vi "BonOMM-SAOMM.Test.vi"() -> ()   [LabVIEW 2011] (continued)
                            n700 = local read "properties.ini"() -> (w3967:path)
                            n701 = call "SerialCommError.vi"("VISA IN"=w3963, "error IN"=w3964) -> ("VISA OUT"=w3978:refnum<visa-resource-name>, "Error"=w3966:bool, "error OUT"=w3958:errorcluster)  [unwired: 11 in]
                            n702 = Not(x=w3966) -> (.not. x?=w3959:bool)
                            n703 = call <vilib>:"Open Config Data.vi"("configuration file path"=w3967) -> ("error out"=w3976:errorcluster, "refnum"=w3977:T24)  [unwired: 8 in, 1 out]
                            n704 = local write "TCS VRN"(w3978) -> ()
                            n705 = local write "TCS Error"(w3958) -> ()
                            n706 = case shown="True" w3959 {
                              tunnel: [TRUE ("Boolean") w4021] -> w3961
                              frame False {
                              }
                              frame True {
                                n707 = Two Button Dialog(message="La connexion TCP/IP semble fonctionner.\nDésirez-vous vraiment la réinitialiser ?" ("T button name (\"OK\")"), 1:"Non" ("F button name (\"Cancel\")"), 2:"Oui" ("T button name (\"OK\")")) -> (T button?=w4021:bool)
                              }
                            }
                            n708 = call-poly <vilib>:"Read Key.vi"("section"=w3971, "error in (no error)"=w3976, "key"="TCS-IP" ("name or relative path"), "refnum"=w3977) -> ("error out"=w3974:errorcluster, "value"=w3962:string, "refnum out"=w3975:T24)  [unwired: 4 in, 1 out]
                            n709 = call-poly <vilib>:"Read Key.vi"("section"=w3971, "error in (no error)"=w3974, "key"="TCS-PN" ("name or relative path"), "refnum"=w3975) -> ("error out"=w3972:errorcluster, "value"=w3968:u32, "refnum out"=w3973:T24)  [unwired: 4 in, 1 out]
                            n710 = call <vilib>:"Close Config Data.vi"("error in (no error)"=w3972, "refnum"=w3973) -> ()  [unwired: 8 in, 2 out]
                            n711 = case shown="True" w3961 {
                              tunnel: w3968 -> [_ w3984]
                              tunnel: w3962 -> [_ w3985]
                              tunnel: w3960 -> [_ w3986]
                              frame False {
                              }
                              frame True {
                                n712 = flat-sequence {
                                tunnel: w3986 -> [w3993]
                                tunnel: [refnum<visa-resource-name> "-1" ("Table VRN")] -> w3981
                                tunnel: [w3990] -> w3980
                                tunnel: w3981 -> [w3997]
                                tunnel: w3980 -> [w3996]
                                tunnel: [w3994] -> w3979
                                tunnel: w3979 -> [_]
                                tunnel: w3985 -> [w4004]
                                tunnel: w3984 -> [w4003]
                                tunnel: [w4002] -> w3983
                                tunnel: [w4001] -> w3982
                                tunnel: [w4015] -> w3988
                                tunnel: [w4014] -> w3987
                                tunnel: w3982 -> [_]
                                tunnel: w3983 -> [w4009]
                                tunnel: w3988 -> [w4017]
                                tunnel: w3987 -> [w4016]
                                frame #0 {
                                w3989 = TRUE ("TCS R actif")
                                n713 = local write "ReconnectionMute"(w3989) -> ()
                                n714 = local read "TCS VRN"() -> (w3990:refnum<visa-resource-name>)
                                n715 = call "TCS-Wait4Flag.vi"("Raise Flag ?"=TRUE, "Ctl Refnum IN"=w3993) -> ()  [unwired: 8 in, 2 out]
                                "TCSMute" <- w3989
                                }
                                frame #1 {
                                n716 = local write "TCS VRN"(w3997) -> ()
                                n717 = Type Cast(type=refnum<k5> refnum ("connection ID out"), x=w3996) -> (*(type *) &x=w3998:refnum<k5>)
                                n718 = TCP Close Connection(connection ID=w3998) -> (error out=w3994:errorcluster)  [unwired: 2 in, 1 out]
                                }
                                frame #2 {
                                n719 = Wait (ms)(milliseconds to wait=u32 1000) -> ()  [unwired: 1 out]
                                }
                                frame #3 {
                                n720 = To Unsigned Word Integer(number=w4003) -> (unsigned 16bit integer=w4005:u16)
                                n721 = local write "TCS actif"(FALSE ("TCS R actif")) -> ()
                                n722 = TCP Open Connection(address=w4004, remote port or service name=w4005) -> (connection ID=w4002:refnum<k5>, error out=w4001:errorcluster)  [unwired: 3 in]
                                }
                                frame #4 {
                                # "Doit-on fermer la \nconnexion d'abord ?"
                                n723 = Type Cast(type="", x=w4009) -> (*(type *) &x=w4012:string)
                                n724 = control-ref of="TCS actif"() -> (w4006:refnum<vi>)
                                n725 = Type Cast(type=refnum<visa-resource-name> "-1" ("Table VRN"), x=w4012) -> (*(type *) &x=w4010:refnum<visa-resource-name>)
                                n726 = call "EXCOM-25-EQ.vi"("VISA resource name"=w4010, "Bool Refnum"=w4006) -> ("VISA resource name dup"=w4008:refnum<visa-resource-name>, "Error OUT"=w4007:errorcluster)  [unwired: 3 in, 13 out]
                                n727 = call "SerialCommError.vi"("VISA IN"=w4008, "error IN"=w4007) -> ("VISA OUT"=w4015:refnum<visa-resource-name>, "error OUT"=w4014:errorcluster)  [unwired: 11 in, 1 out]
                                }
                                frame #5 {
                                n728 = case shown="Error" w4016 {
                                frame No Error {
                                }
                                frame Error {
                                n729 = One Button Dialog(message="La communication avec le TCS ne semble toujours pas foncitonner.\nVérifiez les connexions et les paramètres puis recommencez." ("T button name (\"OK\")")) -> ()  [unwired: 1 in, 1 out]
                                }
                                }
                                n730 = local write "TCS Error"(w4016) -> ()
                                n731 = local write "TCS VRN"(w4017) -> ()
                                }
                                frame #6 {
                                w4019 = FALSE
                                n732 = local write "ReconnectionMute"(w4019) -> ()
                                n733 = local write "TCSMute"(w4019) -> ()
                                }
                                }
                              }
                            }
                          }
                        }
                      }
                      frame "com_Caméra de référence" {
                        n734 = local read "exptime"() -> (w4027:dbl)
                        n735 = local read "MessageType"() -> (w4032:cluster{string[], u32[]})
                        n736 = control-ref of="PrAMS actif"() -> (w4036:refnum<vi>)
                        n737 = local read "Signature"() -> (w4035:u32)
                        n738 = control-ref of="PrAMS-ACK"() -> (w4037:refnum<vi>)
                        n739 = local read "PrAMS VRN"() -> (w4038:refnum<visa-resource-name>)
                        n740 = expression code="x*1000"(w4027) -> (w4030:dbl)
                        n741 = To Unsigned Long Integer(number=w4030) -> (unsigned 32bit integer=w4029:u32)
                        n742 = call-poly "SAOMM-Num2littleEndian.vi"("Number"=w4029) -> ("LiitleEndianedData"=w4028:u8[])  [unwired: 14 in]
                        n743 = call "SAOMM-SendSET.vi"("PRAMMS-COMM IN"=w4038, "Active Refnum"=w4036, "PrAMS-ACK"=w4037, "Signature"=w4035, "Error IN"=errorcluster {"status"=FALSE, "code"=0, "source"=""} ("PRAMMS Error"), "MessageType"=w4032, "Active SET"="emtSetImageExposureTime", "Value (little endianed byte array)"=w4028) -> ("Error"=w4026:bool, "Error OUT"=w4034:errorcluster)  [unwired: 4 in, 2 out]
                        n744 = local write "PrAMS Error"(w4034) -> ()
                        n745 = Not(x=w4026) -> (.not. x?=w4025:bool)
                        n746 = case shown="True" w4025 {
                          tunnel: [TRUE ("Boolean") w4041] -> w4039
                          frame False {
                          }
                          frame True {
                            n747 = Two Button Dialog(message="La connexion TCP/IP semble fonctionner.\nDésirez-vous vraiment la réinitialiser ?" ("T button name (\"OK\")"), 1:"Non" ("F button name (\"Cancel\")"), 2:"Oui" ("T button name (\"OK\")")) -> (T button?=w4041:bool)
                          }
                        }
                        n748 = case shown="True" w4039 {
                          frame False {
                          }
                          frame True {
                            n749 = flat-sequence {
                              tunnel: [w4046] -> w4045
                              tunnel: w4045 -> [_]
                              frame #0 {
                                n750 = local read "PrAMS VRN"() -> (w4048:refnum<visa-resource-name>)
                                n751 = Type Cast(type=refnum<k5> refnum ("connection ID"), x=w4048) -> (*(type *) &x=w4047:refnum<k5>)
                                n752 = TCP Close Connection(connection ID=w4047) -> (error out=w4046:errorcluster)  [unwired: 2 in, 1 out]
                              }
                              frame #1 {
                                n753 = local read "properties.ini"() -> (w4058:path)
                                n754 = local read "path_config"() -> (w4051:path)
                                n755 = Build Path(base path=w4051, name or relative path=path "command.ini" ("command.ini")) -> (appended path=w4050:path)
                                n756 = call <vilib>:"Open Config Data.vi"("create file if necessary (T)"=FALSE, "configuration file path"=w4058) -> ("error out"=w4056:errorcluster, "refnum"=w4055:T24)  [unwired: 7 in, 1 out]
                                n757 = local read "Signature"() -> (w4067:u32)
                                n758 = call-poly <vilib>:"Read Key.vi"("section"="communications" ("key"), "error in (no error)"=w4056, "key"="PRAMMS-IP", "refnum"=w4055) -> ("error out"=w4062:errorcluster, "value"=w4054:string, "refnum out"=w4061:T24)  [unwired: 4 in, 1 out]
                                n759 = call <vilib>:"Close Config Data.vi"("error in (no error)"=w4062, "refnum"=w4061) -> ()  [unwired: 8 in, 2 out]
                                n760 = call "SAOMM-connect.vi"("IP"=w4054, "Port"=u16 10010, "Signature"=w4067, "Command.ini"=w4050) -> ("connection ID"=w4064:refnum<k5>, "Error OUT"=w4053:errorcluster)  [unwired: 7 in, 3 out]
                                n761 = disable-structure shown="Disabled" {
                                disable-tunnel: w4053 -> [w4069 _]
                                frame Disabled {
                                n762 = case shown="Error" w4069 {
                                frame No Error {
                                }
                                frame Error {
                                n763 = One Button Dialog(message="Erreur lors de la connexion\nà l'hexapode-console.") -> ()  [unwired: 1 in, 1 out]
                                }
                                }
                                }
                                frame Enabled {
                                }
                                }
                                n764 = local read "PrAMS VRN"() -> (w4066:refnum<visa-resource-name>)
                                n765 = local write "PrAMS Error"(w4053) -> ()
                                n766 = Type Cast(type=w4054, x=w4064) -> (*(type *) &x=w4063:string)
                                n767 = Type Cast(type=w4066, x=w4063) -> (*(type *) &x=w4065:refnum<visa-resource-name>)
                                n768 = local write "PrAMS VRN"(w4065) -> ()
                              }
                            }
                          }
                        }
                      }
                      frame "com_Tables de guidage" {
                        n769 = flat-sequence {
                          frame #0 {
                            w4072 = TRUE
                            n770 = local write "Sync_Ready"(FALSE ("Sync_Ready")) -> ()
                            "TableMute" <- w4072
                            "ReconnectionMute" <- w4072
                          }
                          frame #1 {
                            w4087 = "communications" ("name or relative path")
                            n771 = local read "Table VRN"() -> (w4076:refnum<visa-resource-name>)
                            n772 = local read "properties.ini"() -> (w4080:path)
                            n773 = control-ref of="Table actif"() -> (w4074:refnum<vi>)
                            n774 = local read "ActiveStages"() -> (w4073:string[])
                            n775 = call "Newmark-Status-All.vi"("Table VRN IN"=w4076, "Bool Refnum"=w4074, "StageTag"=w4073) -> ("Table VRN OUT"=w4077:refnum<visa-resource-name>, "Error OUT"=w4075:errorcluster)  [unwired: 4 in, 11 out]
                            n776 = call <vilib>:"Open Config Data.vi"("configuration file path"=w4080) -> ("error out"=w4092:errorcluster, "refnum"=w4093:T24)  [unwired: 8 in, 1 out]
                            n777 = call "SerialCommError.vi"("VISA IN"=w4077, "error IN"=w4075) -> ("VISA OUT"=w4094:refnum<visa-resource-name>, "Error"=w4078:bool)  [unwired: 11 in, 1 out]
                            n778 = case shown="True" w4078 {
                              selector: w4078 -> [_ w4107]
                              tunnel: [w4103 w4107] -> w4079
                              frame False {
                                n779 = Two Button Dialog(message="La communication avec les tables semble bonne.\nDésirez-vous vraiment le réinitialiser ?" ("T button name (\"OK\")"), 1:"Non" ("F button name (\"Cancel\")"), 2:"Oui" ("T button name (\"OK\")")) -> (T button?=w4103:bool)
                              }
                              frame True {
                              }
                            }
                            n780 = call-poly <vilib>:"Read Key.vi"("section"=w4087, "error in (no error)"=w4092, "key"="tablevrn" ("name or relative path"), "refnum"=w4093) -> ("error out"=w4090:errorcluster, "value"=w4083:string, "refnum out"=w4091:T24)  [unwired: 4 in, 1 out]
                            n781 = local write "Table VRN"(w4094) -> ()
                            n782 = call-poly <vilib>:"Read Key.vi"("section"=w4087, "error in (no error)"=w4090, "key"="tablespd" ("name or relative path"), "refnum"=w4091) -> ("error out"=w4088:errorcluster, "value"=w4084:u32, "refnum out"=w4089:T24)  [unwired: 4 in, 1 out]
                            n783 = Type Cast(type=refnum<visa-resource-name> "-1" ("TCS R VRN"), x=w4083) -> (*(type *) &x=w4081:refnum<visa-resource-name>)
                            n784 = call <vilib>:"Close Config Data.vi"("error in (no error)"=w4088, "refnum"=w4089) -> ()  [unwired: 8 in, 2 out]
                            n785 = case shown="True" w4079 {
                              tunnel: w4084 -> [_ w4100]
                              tunnel: w4081 -> [_ w4099]
                              frame False {
                              }
                              frame True {
                                n786 = local write "Table Baud rate"(w4100) -> ()
                                n787 = control-ref of="Table actif"() -> (w4097:refnum<vi>)
                                n788 = local read "ActiveStages"() -> (w4098:string[])
                                n789 = call "Newmark-Initialize.vi"("VISA resource name"=w4099, "ActiveStages"=w4098, "baud rate"=w4100, "Timeout"=u32 1000, "Bool Refnum"=w4097) -> ("VISA resource name out"=w4101:refnum<visa-resource-name>, "Error OUT"=w4095:errorcluster)  [unwired: 8 in, 1 out]
                                n790 = local write "Table Error"(w4095) -> ()
                                n791 = case shown="No Error" w4095 {
                                frame No Error {
                                }
                                frame Error {
                                n792 = One Button Dialog(message="La communication avec les tables  ne semble toujours pas foncitonner.\nVérifiez les connexions et les paramètres puis recommencez." ("T button name (\"OK\")")) -> ()  [unwired: 1 in, 1 out]
                                }
                                }
                                n793 = local write "Table VRN"(w4101) -> ()
                              }
                            }
                          }
                          frame #2 {
                            w4109 = FALSE
                            n794 = local write "ReconnectionMute"(w4109) -> ()
                            n795 = local write "Sync_Ready"(TRUE ("Sync_Ready")) -> ()
                            n796 = local write "TableMute"(w4109) -> ()
                          }
                        }
                      }
                      frame "com_Secondaire Actif" {
                        (unwired) FALSE
                        w4119 = "communications" ("name or relative path")
                        n797 = local read "properties.ini"() -> (w4114:path)
                        n798 = call <vilib>:"Open Config Data.vi"("configuration file path"=w4114) -> ("error out"=w4124:errorcluster, "refnum"=w4125:T24)  [unwired: 8 in, 1 out]
                        n799 = One Button Dialog(message="À compléter ...") -> ()  [unwired: 1 in, 1 out]
                        n800 = call-poly <vilib>:"Read Key.vi"("section"=w4119, "error in (no error)"=w4124, "key"="PRAMMS-IP" ("name or relative path"), "refnum"=w4125) -> ("error out"=w4122:errorcluster, "value"=w4116:string, "refnum out"=w4123:T24)  [unwired: 4 in, 1 out]
                        n801 = call-poly <vilib>:"Read Key.vi"("section"=w4119, "error in (no error)"=w4122, "key"="PRAMMS-IP" ("name or relative path"), "refnum"=w4123) -> ("error out"=w4120:errorcluster, "value"=w4113:u32, "refnum out"=w4121:T24)  [unwired: 4 in, 1 out]
                        n802 = Type Cast(type=refnum<visa-resource-name> "-1" ("TCS R VRN"), x=w4116) -> (*(type *) &x=w4112:refnum<visa-resource-name>)
                        n803 = call <vilib>:"Close Config Data.vi"("error in (no error)"=w4120, "refnum"=w4121) -> ()  [unwired: 8 in, 2 out]
                        n804 = case shown="True" TRUE {
                          tunnel: w4113 -> [_ _]
                          tunnel: w4112 -> [_ _]
                          frame False {
                          }
                          frame True {
                          }
                        }
                      }
                      frame "com_Lampes de calibration" {
                        n805 = flat-sequence {
                          frame #0 {
                            w4133 = "communications" ("name or relative path")
                            n806 = local read "properties.ini"() -> (w4126:path)
                            n807 = call <vilib>:"Open Config Data.vi"("configuration file path"=w4126) -> ("error out"=w4128:errorcluster, "refnum"=w4127:T24)  [unwired: 8 in, 1 out]
                            n808 = call-poly <vilib>:"Read Key.vi"("section"=w4133, "error in (no error)"=w4128, "key"="calibvrn" ("name or relative path"), "refnum"=w4127) -> ("error out"=w4130:errorcluster, "value"=w4136:string, "refnum out"=w4129:T24)  [unwired: 4 in, 1 out]
                            n809 = call-poly <vilib>:"Read Key.vi"("section"=w4133, "error in (no error)"=w4130, "key"="calibspd" ("name or relative path"), "refnum"=w4129) -> ("error out"=w4132:errorcluster, "value"=w4139:u32, "refnum out"=w4131:T24)  [unwired: 4 in, 1 out]
                            n810 = Type Cast(type=refnum<visa-resource-name> "-1" ("TCS R VRN"), x=w4136) -> (*(type *) &x=w4138:refnum<visa-resource-name>)
                            n811 = call <vilib>:"Close Config Data.vi"("error in (no error)"=w4132, "refnum"=w4131) -> ()  [unwired: 8 in, 2 out]
                            n812 = call-poly "VISA Configure Serial Port"("VISA resource name"=w4138, "timeout (10sec)"=u32 2000, "Enable Termination\nChar (T)"=FALSE ("Enable Termination\nChar (T)"), "baud rate (9600)"=w4139) -> ("VISA resource name out"=w4142:refnum<visa-resource-name>, "error out"=w4143:errorcluster)  [unwired: 10 in]
                            n813 = call "SerialCommError.vi"("VISA IN"=w4142, "error IN"=w4143) -> ("VISA OUT"=w4144:refnum<visa-resource-name>)  [unwired: 11 in, 2 out]
                            n814 = local write "Calib VRN"(w4144) -> ()
                          }
                          frame #1 {
                            n815 = One Button Dialog(message="Le port série des lampes de calibration a été réinitialisé.\n(Aucun test réel car la communication est à sens unique)") -> ()  [unwired: 1 in, 1 out]
                          }
                        }
                      }
                      frame "com_Commandes externes" {
                        (unwired) TRUE
                        n816 = flat-sequence {
                          frame #0 {
                            w4154 = "communications" ("name or relative path")
                            n817 = local read "properties.ini"() -> (w4147:path)
                            n818 = call <vilib>:"Open Config Data.vi"("configuration file path"=w4147) -> ("error out"=w4149:errorcluster, "refnum"=w4148:T24)  [unwired: 8 in, 1 out]
                            n819 = call-poly <vilib>:"Read Key.vi"("section"=w4154, "error in (no error)"=w4149, "key"="excvrn" ("name or relative path"), "refnum"=w4148) -> ("error out"=w4151:errorcluster, "value"=w4157:string, "refnum out"=w4150:T24)  [unwired: 4 in, 1 out]
                            n820 = call-poly <vilib>:"Read Key.vi"("section"=w4154, "error in (no error)"=w4151, "key"="excspd" ("name or relative path"), "refnum"=w4150) -> ("error out"=w4153:errorcluster, "value"=w4160:u32, "refnum out"=w4152:T24)  [unwired: 4 in, 1 out]
                            n821 = Type Cast(type=refnum<visa-resource-name> "-1" ("TCS R VRN"), x=w4157) -> (*(type *) &x=w4159:refnum<visa-resource-name>)
                            n822 = call <vilib>:"Close Config Data.vi"("error in (no error)"=w4153, "refnum"=w4152) -> ()  [unwired: 8 in, 2 out]
                            n823 = call-poly "VISA Configure Serial Port"("VISA resource name"=w4159, "timeout (10sec)"=u32 2000, "Enable Termination\nChar (T)"=FALSE ("Enable Termination\nChar (T)"), "baud rate (9600)"=w4160) -> ("VISA resource name out"=w4163:refnum<visa-resource-name>, "error out"=w4164:errorcluster)  [unwired: 10 in]
                            n824 = call "SerialCommError.vi"("VISA IN"=w4163, "error IN"=w4164) -> ("VISA OUT"=w4146:refnum<visa-resource-name>)  [unwired: 11 in, 2 out]
                            n825 = local write "Excmd VRN"(w4146) -> ()
                          }
                          frame #1 {
                            n826 = One Button Dialog(message="Le port série des communications externes a été réinitialisé.\n(Relancez une commande externe afin de tester la communication)") -> ()  [unwired: 1 in, 1 out]
                          }
                        }
                      }
                      frame "com_MC-BonOMM" {
                        n827 = local read "Périphérique"() -> (w4175:u16)
                        n828 = Two Button Dialog(message="Ceci va redémarrer le contrôleur de roue à filtre\net réinitialiser la communication.\nVoulez-vous continuer ?", 1:"NON" ("F button name (\"Cancel\")"), 2:"OUI" ("T button name (\"OK\")")) -> (T button?=w4166:bool)
                        n829 = Equal?(x=w4175, y=u16 0) -> (x = y?=w4177:bool)
                        n830 = Equal?(x=w4175, y=u16 1) -> (x = y?=w4176:bool)
                        n831 = Equal?(x=w4175, y=u16 2) -> (x = y?=w4178:bool)
                        n832 = Build Array(w4177, w4176, w4178) -> (w4170:bool[])
                        n833 = Boolean Array To Number(Boolean array=w4170) -> (number=w4171:u32)
                        n834 = case shown="True" w4166 {
                          tunnel: w4171 -> [_ w4182]
                          tunnel: [w4179 w4180] -> _
                          frame False {
                            n835 = local read "MC_connect"() -> (w4179:bool)
                          }
                          frame True {
                            n836 = flat-sequence {
                              tunnel: w4182 -> [w4186]
                              tunnel: [w4186] -> w4181
                              tunnel: w4181 -> [w4206]
                              tunnel: [w4192] -> w4180
                              frame #0 {
                                n837 = local read "MC-BonOMM VRN"() -> (w4185:refnum<visa-resource-name>)
                                n838 = flat-sequence {
                                tunnel: w4183 -> [w4190]
                                frame #0 {
                                n839 = Wait (ms)(milliseconds to wait=u32 2000) -> ()  [unwired: 1 out]
                                }
                                frame #1 {
                                n840 = property class="Instr"(reference=w4190) -> (reference out=w4189:refnum<visa-resource-name>, "Serial Settings:Number of Bytes at Serial Port"=w4188:u32)  [unwired: 1 in, 1 out]
                                n841 = local write "MC_connect"(FALSE ("MC_connect")) -> ()
                                n842 = VISA Read(VISA resource name=w4189, byte count=w4188) -> ()  [unwired: 1 in, 4 out]
                                }
                                }
                                n843 = VISA Write(VISA resource name=w4185, write buffer="r" ("Commande")) -> (VISA resource name out=w4183:refnum<visa-resource-name>)  [unwired: 1 in, 2 out]
                              }
                              frame #1 {
                                n844 = local read "MC-BonOMM VRN"() -> (w4202:refnum<visa-resource-name>)
                                n845 = call "MC-BonOMM_talker.vi"("MC-BonOMM VRN"=w4202, "Commande"="m", "byte count"=u32 1, "Timeout (ms)"=2000, "answer=command?"=FALSE) -> ("Answer"=w4196:string, "ok ?"=w4199:bool)
                                n846 = Equal?(x="f", y=w4196) -> (x = y?=w4195:bool)
                                n847 = Equal?(x=w4196, y="x") -> (x = y?=w4194:bool)
                                n848 = Or(x=w4195, y=w4194) -> (x .or. y?=w4193:bool)
                                n849 = And(x=w4193, y=w4199) -> (x .and. y?=w4200:bool)
                                n850 = case shown="True" w4200 {
                                tunnel: w4206 -> [_ w4212]
                                tunnel: [w4207 w4211] -> w4192
                                frame False {
                                n851 = One Button Dialog(message="Problème de communication avec MC-BonOMM", button name ("OK")="Oups :(") -> (true=w4208:bool)
                                n852 = Not(x=w4208) -> (.not. x?=w4207:bool)
                                }
                                frame True {
                                n853 = stacked-sequence {
                                tunnel: w4212 -> [w4214 w4225]
                                tunnel: [_ w4223] -> w4211
                                frame #0 {
                                n854 = case shown="1, Default" w4214 {
                                tunnel: ["f" "o" "x"] -> w4213
                                frame 1, Default {
                                }
                                frame 2 {
                                }
                                frame 4 {
                                }
                                }
                                n855 = local read "MC-BonOMM VRN"() -> (w4217:refnum<visa-resource-name>)
                                n856 = call "MC-BonOMM_talker.vi"("MC-BonOMM VRN"=w4217, "Commande"=w4213, "Timeout (ms)"=2000, "answer=command?"=TRUE) -> ("ok ?"=w4215:bool)  [unwired: 1 in, 1 out]
                                n857 = case shown="False" w4215 {
                                frame False {
                                n858 = One Button Dialog(message="Erreur lors du changement de mode ...") -> ()  [unwired: 1 in, 1 out]
                                }
                                frame True {
                                }
                                }
                                n859 = local write "MC_connect"(w4215) -> ()
                                }
                                frame #1 {
                                n860 = local read "MC-BonOMM VRN"() -> (w4224:refnum<visa-resource-name>)
                                n861 = case shown="1, 2, Default" w4225 {
                                tunnel: w4224 -> [w4231 w4241]
                                tunnel: [w4229 w4240] -> w4223
                                frame 1, 2, Default {
                                n862 = call "MC-BonOMM_talker.vi"("MC-BonOMM VRN"=w4231, "Commande"="q", "byte count"=u32 1, "Timeout (ms)"=8000, "answer=command?"=FALSE) -> ("Answer"=w4230:string, "ok ?"=w4229:bool)
                                n863 = Decimal String To Number(string=w4230) -> (number=w4234:i32)  [unwired: 2 in, 1 out]
                                n864 = local write "F#"(w4234) -> ()
                                n865 = case shown="1..6" w4234 {
                                selector: w4234 -> [w4236 _]
                                tunnel: [w4235 ""] -> w4233
                                frame 1..6 {
                                n866 = local read "Tableau des filtres"() -> (w4237:string[])
                                n867 = Decrement(x=w4236) -> (x-1=w4238:i32)
                                n868 = Index Array(array=w4237, index=w4238) -> (element=w4235:string)
                                }
                                frame 0, Default {
                                }
                                }
                                n869 = local write "filtre_nom"(w4233) -> ()
                                }
                                frame 4 {
                                n870 = local read "ST_SPD"() -> (w4242:dbl)
                                n871 = call "Change_speed.vi"("ST_SPD"=w4242, "MC-BonOMM VRN"=w4241) -> ("Connected?"=w4240:bool)
                                n872 = case shown="False" w4240 {
                                frame False {
                                n873 = property on="Périphérique" class="Ring (strict)"("Value (Signaling)"=u16 3) -> ()  [unwired: 2 in, 2 out]
                                }
                                frame True {
                                }
                                }
                                }
                                }
                                }
                                }
                                }
                                }
                                n874 = local write "MC_connect"(w4192) -> ()
                              }
                            }
                          }
                        }
                      }
                      frame "com_Station Météo" {
                        # "Réinitialisation de la connexion avec le cRIO de météo"
                        n875 = flat-sequence {
                          tunnel: [w4250] -> w4245
                          tunnel: w4245 -> [w4268]
                          tunnel: [w4268] -> w4244
                          frame #0 {
                            # "Ferme la connexion si elle est ouverte"
                            n876 = local read "Cx"() -> (w4246:bool)
                            n877 = case shown="True" w4246 {
                              frame False {
                              }
                              frame True {
                                n878 = local read "cRIO_commID"() -> (w4247:refnum<k5>)
                                n879 = TCP Close Connection(connection ID=w4247) -> ()  [unwired: 2 in, 2 out]
                              }
                            }
                          }
                          frame #1 {
                            n880 = local read "cRIO Port"() -> (w4248:u16)
                            n881 = local read "cRIO address"() -> (w4254:string)
                            n882 = TCP Open Connection(address=w4254, remote port or service name=w4248) -> (connection ID=w4255:refnum<k5>, error out=w4252:errorcluster)  [unwired: 3 in]
                            n883 = Unbundle By Name(w4252) -> ("status"=w4253:bool)
                            n884 = local write "cRIO_commID"(w4255) -> ()
                            n885 = Not(x=w4253) -> (.not. x?=w4249:bool)
                            n886 = local write "Cx"(w4249) -> ()
                            n887 = case shown="True" w4249 {
                              tunnel: [errorcluster {"status"=FALSE, "code"=0, "source"=""} ("error out") w4258] -> w4251
                              frame False {
                                w4257 = 0.0 ("indic-T-out")
                                n888 = local write "indic-Tm"(w4257) -> ()
                                n889 = local write "indic-T-struct"(w4257) -> ()
                                n890 = local write "indic-T-out"(w4257) -> ()
                                n891 = local write "indic-T-in"(w4257) -> ()
                                n892 = local write "indic-H-out"(w4257) -> ()
                                n893 = local write "indic-H-in"(w4257) -> ()
                              }
                              frame True {
                                n894 = local read "cRIO_commID"() -> (w4266:refnum<k5>)
                                n895 = call "TCP-read.vi"("connection ID"=w4266) -> ("error out"=w4258:errorcluster, "data out"=w4267:string)  [unwired: 2 in, 1 out]
                                n896 = call "line2array.vi"("data-line"=w4267) -> ("data-array"=w4265:dbl[])  [unwired: 2 out]
                                n897 = Index Array(array=w4265) -> (element #1=w4264:dbl, element #2=w4263:dbl, element #3=w4262:dbl, element #4=w4261:dbl, element #7=w4260:dbl, element #8=w4259:dbl)  [unwired: 9 in, 3 out]
                                n898 = local write "indic-Tm"(w4260) -> ()
                                n899 = local write "indic-T-struct"(w4259) -> ()
                                n900 = local write "indic-T-out"(w4264) -> ()
                                n901 = local write "indic-T-in"(w4262) -> ()
                                n902 = local write "indic-H-out"(w4263) -> ()
                                n903 = local write "indic-H-in"(w4261) -> ()
                              }
                            }
                            n904 = Unbundle By Name(w4251) -> ("status"=w4250:bool)
                          }
                          frame #2 {
                            n905 = case shown="True" w4268 {
                              frame False {
                              }
                              frame True {
                                n906 = One Button Dialog(message="La communication avec la station météo n'a pu être rétablie.\nVérifier les connexions réseaux ou redémarrer le système.") -> ()  [unwired: 1 in, 1 out]
                              }
                            }
                          }
                        }
                        n907 = Not(x=w4244) -> ()  [unwired: 1 out]
                      }
                      frame "com_Caméra de guidage" {
                        (unwired) FALSE ("Boolean")
                      }
                      frame "com_Reconnexion automatique ?" {
                        n908 = local read "AutoConnect?"() -> (w4271:bool)
                        n909 = Not(x=w4271) -> (.not. x?=→"AutoConnect?":bool)
                      }
                    }
                  }
                  frame "main_Instruments" {
                    # "Ajouter le charement de la LUT approprié ..."
                    n910 = String Subset(string=w4274, offset (0)=4) -> (substring=w4273:string)  [unwired: 1 in]
                    n911 = local read "Instrument Actuel"() -> (w4275:string)
                    n912 = Not Equal?(x=w4273, y=w4275) -> (x != y?=w4276:bool)
                    n913 = case shown="True" w4276 {
                      tunnel: w4273 -> [_ w4291]
                      tunnel: w4275 -> [_ w4287]
                      frame False {
                      }
                      frame True {
                        n914 = local read "instruments.ini"() -> (w4292:path)
                        n915 = Current VI's Menubar() -> (w4290:refnum<k9>)
                        n916 = Set Menu Item Info(6:FALSE ("checked"), 7:w4287, 11:w4290) -> (0:w4288:errorcluster, 3:w4289:refnum<k9>)  [unwired: 4 in]
                        n917 = call "InstrChoice.vi"("Instrument IN"=w4291, "instruments.ini"=w4292, "DisallowUndo"=FALSE) -> ("Modifier?"=w4277:bool, "Instrument OUT"=w4284:string, "FoV"=w4282:dbl, "foynom"=w4283:i32, "atherm"=w4281:dbl, "exclusion"=w4280:path, "collim"=w4279:path)  [unwired: 9 in, 1 out]
                        n918 = Set Menu Item Info(6:TRUE ("checked"), 7:w4284, 8:w4288, 11:w4289) -> ()  [unwired: 3 in, 2 out]
                        n919 = case shown="True" w4277 {
                          tunnel: w4284 -> [_ w4304]
                          tunnel: w4283 -> [_ w4303]
                          tunnel: w4282 -> [_ w4302]
                          tunnel: w4281 -> [_ w4301]
                          tunnel: w4280 -> [_ w4300]
                          tunnel: w4279 -> [_ w4294]
                          frame False {
                          }
                          frame True {
                            n920 = local write "Instrument Actuel"(w4304) -> ()
                            n921 = local write "path_exclusion"(w4300) -> ()
                            n922 = local write "FOV"(w4302) -> ()
                            n923 = local write "Foyer à 0°"(w4303) -> ()
                            n924 = local write "Ath_coef"(w4301) -> ()
                            n925 = local write "ActiveLUT"(w4294) -> ()
                            n926 = call "SAOMM-XML2LUT.vi"("Path"=w4294) -> ("NominalPositions"=w4293:dbl[])  [unwired: 13 in, 1 out]
                            n927 = Index Array(array=w4293) -> (element #3=w4299:dbl, element #4=w4298:dbl, element #5=w4297:dbl, element #6=w4296:dbl, element #7=w4295:dbl)  [unwired: 7 in, 2 out]
                            n928 = local write "Nominal Y"(w4298) -> ()
                            n929 = local write "Nominal X"(w4299) -> ()
                            n930 = local write "Nominal Z"(w4297) -> ()
                            n931 = local write "Nominal V"(w4295) -> ()
                            n932 = local write "Nominal U"(w4296) -> ()
                          }
                        }
                      }
                    }
                  }
                  frame "main_Scripts et Automatismes" {
                    n933 = case shown="\"scp_Charger la librairie de la queue\"" w4305 {
                      selector: w4305 -> [w4309 _ _ _ _ _]
                      frame "", Default {
                        n934 = Concatenate Strings("Erreur avec le menu, cela ne devrait pas se produire ...\nCommande : (\"" ("message"), w4309, "\")" ("message")) -> (w4307:string)
                        n935 = One Button Dialog(message=w4307) -> ()  [unwired: 1 in, 1 out]
                      }
                      frame "scp_Charger la librairie de la queue" {
                        n936 = local read "properties.ini"() -> (w4310:path)
                        n937 = local read "path_libdir"() -> (w4313:path)
                        n938 = call "Get_properties.vi"("Keyword"="queuelib" ("Section"), "Section"="chemins", "properties.ini"=w4310) -> ("error"=w4314:bool, "string"=w4312:string)  [unwired: 6 in, 1 out]
                        n939 = case shown="False" w4314 {
                          tunnel: w4313 -> [w4320 _]
                          tunnel: w4312 -> [w4329 _]
                          tunnel: "table_technicien.dat" -> [w4326 _]
                          frame False {
                            n940 = Build Path(base path=w4320, name or relative path=w4326) -> (appended path=w4325:path)
                            n941 = File/Directory Info(path=w4325) -> (path out=w4322:path, error out=w4324:errorcluster)  [unwired: 1 in, 5 out]
                            n942 = Unbundle By Name(w4324) -> ("status"=w4323:bool)
                            n943 = local read "wgetexec"() -> (w4327:path)
                            n944 = case shown="False" w4323 {
                              tunnel: w4322 -> [w4352 w4354]
                              tunnel: [w4351 w4354] -> w4321
                              tunnel: w4320 -> [w4350 w4353]
                              tunnel: [w4350 w4353] -> w4319
                              frame False {
                                n945 = Delete(path (use dialog)=w4352) -> (deleted path=w4351:path)  [unwired: 4 in, 2 out]
                              }
                              frame True {
                              }
                            }
                            n946 = Path To String(path=w4327) -> (string=w4317:string)
                            n947 = Concatenate Strings(w4317, " --http-user=carpe", " --http-password=noctem ", w4329) -> (w4332:string)
                            n948 = call <vilib>:"System Exec.vi"("run minimized? (F)"=TRUE, "working directory"=w4319, "command line"=w4332) -> ("error out"=w4318:errorcluster)  [unwired: 5 in, 3 out]
                            n949 = flat-sequence {
                              tunnel: w4321 -> [w4336]
                              tunnel: w4318 -> [w4333]
                              frame #0 {
                                n950 = local write "wget error"(w4333) -> ()
                                n951 = call "Read_obs_files.vi"("Path"=w4336) -> ("path used"=w4334:path, "Output Table"=w4338:string[][])
                                n952 = local read "LST"() -> (w4337:dbl)
                                n953 = for {
                                tunnel: w4338 -> [w4344] mode=indexing
                                tunnel: w4337 -> [w4345]
                                tunnel: [w4341] -> w4335 mode=indexing
                                n954 = Index Array(array=w4344, index #1=2 ("index"), index #2=3 ("index")) -> (element #1=w4347:string, element #2=w4346:string)
                                n955 = call "Airmass.vi"("temps sidéral"=w4345, "DEC"=w4346, "RA"=w4347) -> ("airmass"=w4342:dbl)
                                n956 = Number To Fractional String(number=w4342, precision (6)=i16 2) -> (F-format string=w4343:string)  [unwired: 2 in]
                                n957 = Insert Into Array(array=w4344, index=5, new element=w4343) -> (w4341:string[])
                                }
                                n958 = local write "loaded_lib"(w4334) -> ()
                                n959 = local write "Librairie des objets"(w4335) -> ()
                                n960 = local write "Librairie complète"(w4335) -> ()
                              }
                            }
                          }
                          frame True {
                          }
                        }
                      }
                      frame "scp_Charger une libraire d'objets" {
                        # "Chemin à confirmer,\nvoir avec Mr Turbide ..."
                        # "Gestion du menu en développement ..."
                        n961 = local read "path_libdir"() -> (w4355:path)
                        n962 = File Dialog(6:"*.txt" ("pattern"), 7:"Sélectionner la libraire désirée ..." ("prompt"), 11:w4355) -> (0:w4356:errorcluster, 2:w4360:bool, 3:w4357:path)  [unwired: 4 in, 1 out]
                        n963 = Unbundle(w4356) -> ()  [unwired: 3 out]
                        n964 = case shown="True" w4360 {
                          tunnel: w4357 -> [_ w4366]
                          frame False {
                          }
                          frame True {
                            n965 = local write "loaded_lib"(w4366) -> ()
                            n966 = local read "LST"() -> (w4363:dbl)
                            n967 = call "Read_obs_files.vi"("Path"=w4366) -> ("Output Table"=w4371:string[][])  [unwired: 1 out]
                            n968 = Strip Path(path=w4366) -> (stripped path=w4365:path)  [unwired: 1 out]
                            n969 = for {
                              tunnel: w4371 -> [w4377] mode=indexing
                              tunnel: w4363 -> [w4378]
                              tunnel: [w4374] -> w4362 mode=indexing
                              n970 = Index Array(array=w4377, index #1=2 ("index"), index #2=3 ("index")) -> (element #1=w4380:string, element #2=w4379:string)
                              n971 = call "Airmass.vi"("temps sidéral"=w4378, "DEC"=w4379, "RA"=w4380) -> ("airmass"=w4375:dbl)
                              n972 = Number To Fractional String(number=w4375, precision (6)=i16 2) -> (F-format string=w4376:string)  [unwired: 2 in]
                              n973 = Insert Into Array(array=w4377, index=5, new element=w4376) -> (w4374:string[])
                            }
                            n974 = Path To String(path=w4365) -> (string=w4367:string)
                            n975 = local write "Librairie des objets"(w4362) -> ()
                            n976 = control-ref of="TERMINAL"() -> (w4364:refnum<vi>)
                            n977 = control-ref of="Indicateur d'état"() -> (w4361:refnum<vi>)
                            n978 = Concatenate Strings("Chargement de la librairie \"", w4367, "\"") -> (w4370:string)
                            n979 = call "TERMINAL.vi"("Indicateur Refnum"=w4361, "Terminal Refnum"=w4364, "Indicateur d'état"=w4370) -> ()
                          }
                        }
                      }
                      frame "scp_Modifier la liste des filtres" {
                        n980 = call "ChoixFiltres.vi"("Ordre des filtres Avant"="Tableau des filtres") -> ("Ordre des filtres Après"=w4383:string[])
                        n981 = local write "Tableau des filtres"(w4383) -> ()
                      }
                      frame "scp_Calibration du foyer automatique" {
                        # "À refaire avec le nouveau détecteur ..."
                      }
                      frame "scp_Calibration du champ" {
                        n982 = local read "CentreTel X"() -> (w4388:dbl)
                        n983 = local read "CentreTel Y"() -> (w4387:dbl)
                        n984 = local read "Reference X"() -> (w4386:dbl)
                        n985 = local read "Reference Y"() -> (w4385:dbl)
                        n986 = local read "TableAstrom"() -> (w4390:T4)
                        n987 = call "Starast.vi"("Ry"=w4385, "Rx"=w4386, "Centre Y"=w4387, "Centre X"=w4388, "Table Astrometry IN"=w4390) -> ("Table Astrometry OUT"=w4389:T4)  [unwired: 6 in]
                        n988 = local write "TableAstrom"(w4389) -> ()
                      }
                    }
                  }
                  frame "main_Télescope" {
                    n989 = case shown="\"tel_Synchroniser les horloges\"" w4391 {
                      frame Default {
                      }
                      frame "tel_Synchroniser la coupole" {
                        n990 = stacked-sequence {
                          frame #0 {
                            n991 = control-ref of="TERMINAL"() -> (w4394:refnum<vi>)
                            n992 = control-ref of="Indicateur d'état"() -> (w4393:refnum<vi>)
                            n993 = call "TERMINAL.vi"("Indicateur Refnum"=w4393, "Terminal Refnum"=w4394, "Indicateur d'état"="Synchronisation de la coupole sur la position du télescope") -> ()
                          }
                          frame #1 {
                            # "Synchronise la coupole a la \nposition du télescope"
                            n994 = control-ref of="TCS actif"() -> (w4395:refnum<vi>)
                            n995 = local read "TCS VRN"() -> (w4402:refnum<visa-resource-name>)
                            n996 = Build Array(0.0 ("string1")) -> (w4400:dbl[])
                            n997 = call "EXCOM-CMD.vi"("VRN IN"=w4402, "Bool Refnum"=w4395, "Commande #"=2, "Args"=w4400) -> ("VRN OUT"=w4398:refnum<visa-resource-name>, "OK Done"=w4397:bool, "Error OUT"=w4396:errorcluster)  [unwired: 9 in]
                            n998 = local write "TCS Error"(w4396) -> ()
                            n999 = local write "TCS VRN"(w4398) -> ()
                            n1000 = case shown="False" w4397 {
                              frame False {
                                n1001 = One Button Dialog(message="ATTENTION!!\nLa commande de synchronisation de la coupole a échouée.\nVérifiez la communication avec TCS et recommencez.", button name ("OK")="OK" ("nom du bouton (\"OK\")")) -> ()  [unwired: 1 out]
                              }
                              frame True {
                              }
                            }
                          }
                        }
                      }
                      frame "tel_Synchroniser les horloges" {
                        n1002 = stacked-sequence {
                          seq-local: [w4408 _ _ _] -> [_ _ _ w4426]
                          frame #0 {
                            n1003 = local read "Epoch Tel"() -> (w4408:dbl)
                          }
                          frame #1 {
                            # "Initialise TCS"
                            n1004 = call "GetUTC.vi"() -> ("UTC_fractional"=w4418:dbl, "Day"=w4417:dbl, "Month"=w4416:dbl, "Year"=w4415:dbl, "DST?"=→"DST?":bool)  [unwired: 4 out]
                            n1005 = control-ref of="TCS actif"() -> (w4409:refnum<vi>)
                            n1006 = local read "TCS VRN"() -> (w4420:refnum<visa-resource-name>)
                            n1007 = Build Array(w4415, w4416, w4417, w4418) -> (w4414:dbl[])
                            n1008 = call "EXCOM-CMD.vi"("VRN IN"=w4420, "Bool Refnum"=w4409, "Commande #"=1, "Args"=w4414) -> ("VRN OUT"=w4413:refnum<visa-resource-name>, "OK Done"=w4412:bool, "Error OUT"=w4411:errorcluster)  [unwired: 9 in]
                            n1009 = local write "TCS Error"(w4411) -> ()
                            n1010 = local write "TCS VRN"(w4413) -> ()
                            n1011 = case shown="True" w4412 {
                              frame False {
                                n1012 = One Button Dialog(message="ATTENTION!!\nLa commande INITIALISE TCS\na échoué.\nVérifiez TCS.", button name ("OK")="OK" ("nom du bouton (\"OK\")")) -> ()  [unwired: 1 out]
                              }
                              frame True {
                                n1013 = Wait (ms)(milliseconds to wait=u32 10 ("attente (ms)")) -> ()  [unwired: 1 out]
                              }
                            }
                          }
                          frame #2 {
                            n1014 = Wait (ms)(milliseconds to wait=u32 250) -> ()  [unwired: 1 out]
                          }
                          frame #3 {
                            n1015 = control-ref of="TCS actif"() -> (w4425:refnum<vi>)
                            n1016 = local read "TCS VRN"() -> (w4428:refnum<visa-resource-name>)
                            n1017 = Build Array(w4426) -> (w4431:dbl[])
                            n1018 = call "EXCOM-CMD.vi"("VRN IN"=w4428, "Bool Refnum"=w4425, "Commande #"=22, "Args"=w4431) -> ("VRN OUT"=w4429:refnum<visa-resource-name>, "Error OUT"=w4427:errorcluster)  [unwired: 9 in, 1 out]
                            n1019 = local write "TCS VRN"(w4429) -> ()
                            n1020 = local write "TCS Error"(w4427) -> ()
                          }
                        }
                        n1021 = control-ref of="TERMINAL"() -> (w4407:refnum<vi>)
                        n1022 = control-ref of="Indicateur d'état"() -> (w4406:refnum<vi>)
                        n1023 = call "TERMINAL.vi"("Indicateur Refnum"=w4406, "Terminal Refnum"=w4407, "Indicateur d'état"="Commande d'initialisation de TCS") -> ()
                      }
                      frame "tel_Modifier la vitesse du télescope" {
                        # "Changer la vitesse"
                        n1024 = control-ref of="TCS actif"() -> (w4432:refnum<vi>)
                        n1025 = local read "TCS VRN"() -> (w4436:refnum<visa-resource-name>)
                        n1026 = local read "TCS Error"() -> (w4434:errorcluster)
                        n1027 = control-ref of="TERMINAL"() -> (w4439:refnum<vi>)
                        n1028 = control-ref of="Indicateur d'état"() -> (w4440:refnum<vi>)
                        n1029 = call "Set speed.vi"("VRN IN"=w4436, "Bool Refnum"=w4432, "error IN"=w4434) -> ("VRN OUT"=w4435:refnum<visa-resource-name>, "OK Done"=w4437:bool, "error out"=w4433:errorcluster)  [unwired: 10 in]
                        n1030 = local write "TCS VRN"(w4435) -> ()
                        n1031 = local write "TCS Error"(w4433) -> ()
                        n1032 = call "TERMINAL.vi"("Indicateur Refnum"=w4440, "Terminal Refnum"=w4439, "Indicateur d'état"="Commande de changement des vitesse de TCS") -> ()
                        n1033 = case shown="False" w4437 {
                          frame False {
                            n1034 = One Button Dialog(message="ATTENTION!!\nLa commande CHANGER VITESSE a échoué.\nVérifiez TCS.", button name ("OK")="OK" ("nom du bouton (\"OK\")")) -> ()  [unwired: 1 out]
                          }
                          frame True {
                          }
                        }
                      }
                      frame "tel_Modifier la vitesse de guidage" {
                        n1035 = local read "RateRA"() -> (w4447:dbl)
                        n1036 = expression code="1000/x"(w4447) -> (w4446:dbl)
                        n1037 = call "GuideRate.vi"("Guide Rate"=w4446) -> ("Guide Rate out"=w4444:dbl)  [unwired: 14 in]
                        n1038 = Build Array(w4444) -> (w4445:dbl[])
                        n1039 = expression code="1000/x"(w4444) -> (w4443:dbl)
                        n1040 = control-ref of="TCS actif"() -> (w4450:refnum<vi>)
                        n1041 = local read "TCS VRN"() -> (w4451:refnum<visa-resource-name>)
                        n1042 = call "EXCOM-CMD.vi"("VRN IN"=w4451, "Bool Refnum"=w4450, "Commande #"=15, "Args"=w4445) -> ("VRN OUT"=w4452:refnum<visa-resource-name>, "Error OUT"=w4448:errorcluster)  [unwired: 9 in, 1 out]
                        n1043 = local write "RateDEC"(w4443) -> ()
                        n1044 = local write "RateRA"(w4443) -> ()
                        n1045 = local write "TCS Error"(w4448) -> ()
                        n1046 = local write "TCS VRN"(w4452) -> ()
                      }
                      frame "tel_Modifier l'époque d'affichage" {
                        # "Ne change pas l'équinoxe de TCS mais seulement l'affichage pour BonOMM"
                        n1047 = local read "Epoch Tel"() -> (w4454:dbl)
                        n1048 = local read "AnnéeRL"() -> (w4455:dbl)
                        n1049 = call "Set_epoch.vi"("AnnéeRL"=w4455, "EPOCH_AFF"=w4454) -> ("EPOCH_OUT"=w4453:dbl)
                        n1050 = local write "dflt-EQX"(w4453) -> ()
                        n1051 = disable-structure shown="Disabled" {
                          disable-tunnel: w4453 -> [w4456 _]
                          frame Disabled {
                            n1052 = control-ref of="TCS actif"() -> (w4457:refnum<vi>)
                            n1053 = local read "TCS VRN"() -> (w4463:refnum<visa-resource-name>)
                            n1054 = Build Array(w4456) -> (w4458:dbl[])
                            n1055 = call "EXCOM-CMD.vi"("VRN IN"=w4463, "Bool Refnum"=w4457, "Commande #"=22 ("NombredArguments"), "Args"=w4458) -> ("VRN OUT"=w4461:refnum<visa-resource-name>, "OK Done"=w4459:bool, "Error OUT"=w4460:errorcluster)  [unwired: 9 in]
                            n1056 = local write "TCS Error"(w4460) -> ()
                            n1057 = local write "TCS VRN"(w4461) -> ()
                            n1058 = case shown="False" w4459 {
                              frame False {
                                n1059 = One Button Dialog(message="Erreur lors du chargement de la nouvelle époque d'affichage.\nVérifier la communication avec TCS et recommencez.") -> ()  [unwired: 1 in, 1 out]
                              }
                              frame True {
                              }
                            }
                          }
                          frame Enabled {
                          }
                        }
                      }
                      frame "tel_Reconnexion" {
                        n1060 = One Button Dialog(message="Devrait reconnecter TCS ...") -> ()  [unwired: 1 in, 1 out]
                      }
                    }
                  }
                  frame "main_Secondaire Actif" {
                    n1061 = case shown="\"hex_Panneau de offset\"" w4466 {
                      frame Default {
                      }
                      frame "hex_Commander l'hexapode" {
                        n1062 = flat-sequence {
                          frame #0 {
                            "HexaSpam" <- TRUE ("HexaSpam")
                          }
                          frame #1 {
                            # "Attention, erreur d'époque possible ..."
                            n1063 = disable-structure shown="Enabled" {
                              frame Disabled {
                                # "Rafraichi la position de l'hexapode 2x par seconde"
                                n1064 = local read "Hexapod VRN"() -> (w4484:refnum<visa-resource-name>)
                                n1065 = local read "MessageType"() -> (w4485:cluster{string[], u32[]})
                                n1066 = local read "PrAMS VRN"() -> (w4487:refnum<visa-resource-name>)
                                n1067 = control-ref of="HexX"() -> (w4470:refnum<vi>)
                                n1068 = control-ref of="HexY"() -> (w4471:refnum<vi>)
                                n1069 = control-ref of="HexZ"() -> (w4472:refnum<vi>)
                                n1070 = control-ref of="HexU"() -> (w4473:refnum<vi>)
                                n1071 = control-ref of="HexV"() -> (w4474:refnum<vi>)
                                n1072 = local read "Signature"() -> (w4486:u32)
                                n1073 = Bundle("PrAMS VRN"=w4487, "Signature"=w4486, "MessageType"=w4485, "Hexapod VRN"=w4484) -> (w4483:T27)  [unwired: 1 in]
                                n1074 = Bundle("HexX"=w4470, "HexY"=w4471, "HexZ"=w4472, "HexU"=w4473, "HexV"=w4474) -> (w4469:T28)  [unwired: 1 in]
                                n1075 = control-ref of="Angle Hor."() -> (w4477:refnum<vi>)
                                n1076 = control-ref of="DEC Tel"() -> (w4476:refnum<vi>)
                                n1077 = control-ref of="PrAMS-ACK"() -> (w4479:refnum<vi>)
                                n1078 = control-ref of="Hexapod-ACK"() -> (w4481:refnum<vi>)
                                n1079 = control-ref of="Epoch Tel"() -> (w4468:refnum<vi>)
                                n1080 = control-ref of="PrAMS actif"() -> (w4482:refnum<vi>)
                                n1081 = control-ref of="HexaCons actif"() -> (w4480:refnum<vi>)
